vi "format set pattern.vi"(8 "error in (no error)":errorcluster, 10 "pattern":u8, 11 "format":u32) -> (0 "error out":errorcluster)   [LabVIEW 8.6]
doc: "void format_set_pattern(lxw_format format, uint8_t pattern);"
uses:
  pending_lvxlsxwriter/xlsxwriter.dll
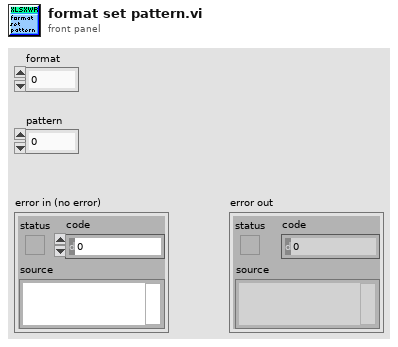
[diagram p1: front panel]
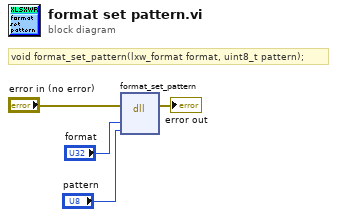
[diagram p0: block diagram]
diagram:
  # "void format_set_pattern(lxw_format format, uint8_t pattern);"
  n1 = dll-call lib="C:/Users/WDAGUtilityAccount/Desktop/pending_lvxlsxwriter/xlsxwriter.*" fn="format_set_pattern"(error in="error in (no error)", "format"="format", "pattern"="pattern") -> (error out=→"error out":errorcluster)  [unwired: 5 in, 1 out]
